vi "CAN Get Error Text.vi"(8 "error in (no error)":errorcluster, 9 "Buffer":string, 10 "Language":u16, 11 "Error":u32) -> (0 "error out":errorcluster, 1 "Buffer out":string, 3 "function return":u32)   [LabVIEW 2025, in "PCAN2023.lvlib"]
doc: "Returns a descriptive text of a given TPCANStatus error code, in any desired language\n\nTPCANStatus __stdcall CAN_GetErrorText(\n TPCANStatus Error, \n WORD Language, \n LPSTR Buffer);"
uses:
  PCAN2023.lvlib
  x64/PCANBasic.dll
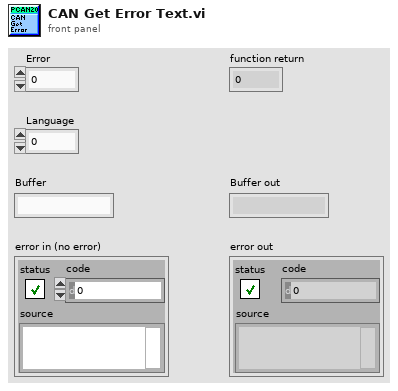
[diagram p1: front panel]
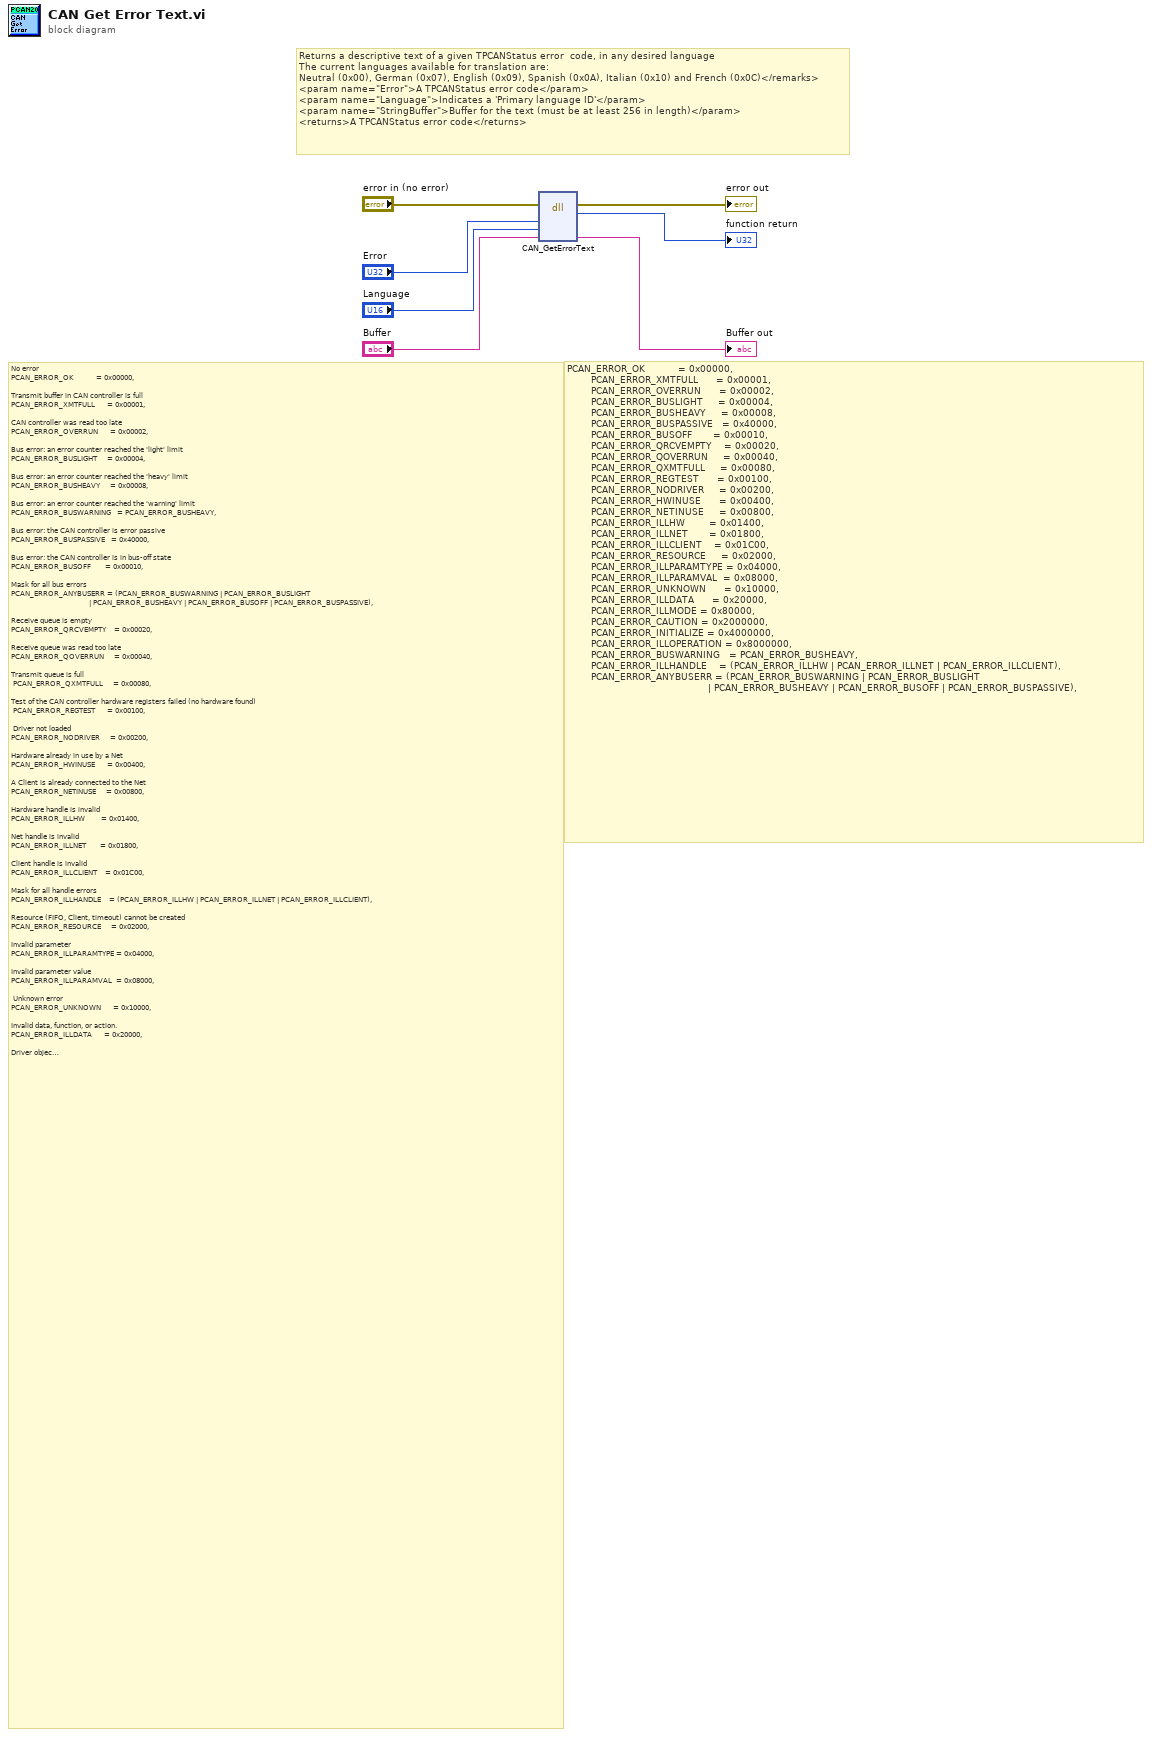
[diagram p0: block diagram]
diagram:
  # "PCAN_ERROR_OK           = 0x00000,\n        PCAN_ERROR_XMTFULL      = 0x00001,\n        PCAN_ERROR_OVERRUN      = 0x00002,  \n        PCAN_ERROR_BUSLIGHT     = 0x00004,  \n        PCAN_ERROR_BUSHEAVY     = 0x00008,  \n        PCAN_ERROR_BUSPASSIVE   = 0x40000,\n        PCAN_ERROR_BUSOFF       = 0x00010,  \n        PCAN_ERROR_QRCVEMPTY    = 0x00020,  \n        PCAN_ERROR_QOVERRUN     = 0x00040,  \n        PCAN_ERROR_QXMTFULL     = 0x00080,  \n        PCAN_ERROR_REGTEST      = 0x00100,\n        PCAN_ERROR_NODRIVER     = 0x00200,\n        PCAN_ERROR_HWINUSE      = 0x00400,\n        PCAN_ERROR_NETINUSE     = 0x00800,\n        PCAN_ERROR_ILLHW        = 0x01400,\n        PCAN_ERROR_ILLNET       = 0x01800,\n        PCAN_ERROR_ILLCLIENT    = 0x01C00,\n        PCAN_ERROR_RESOURCE     = 0x02000,\n        PCAN_ERROR_ILLPARAMTYPE = 0x04000,\n        PCAN_ERROR_ILLPARAMVAL  = 0x08000,\n        PCAN_ERROR_UNKNOWN      = 0x10000,\n        PCAN_ERROR_ILLDATA      = 0x20000,\n        PCAN_ERROR_ILLMODE = 0x80000,\n        PCAN_ERROR_CAUTION = 0x2000000,\n        PCAN_ERROR_INITIALIZE = 0x4000000,\n        PCAN_ERROR_ILLOPERATION = 0x8000000,\n        PCAN_ERROR_BUSWARNING   = PCAN_ERROR_BUSHEAVY,\n        PCAN_ERROR_ILLHANDLE    = (PCAN_ERROR_ILLHW | PCAN_ERROR_ILLNET | PCAN_ERROR_ILLCLIENT),\n        PCAN_ERROR_ANYBUSERR = (PCAN_ERROR_BUSWARNING | PCAN_ERROR_BUSLIGHT \n                                               | PCAN_ERROR_BUSHEAVY | PCAN_ERROR_BUSOFF | PCAN_ERROR_BUSPASSIVE),"
  # "No error\nPCAN_ERROR_OK           = 0x00000,\n\nTransmit buffer in CAN controller is full\nPCAN_ERROR_XMTFULL      = 0x00001,\n\nCAN controller was read too late        \nPCAN_ERROR_OVERRUN      = 0x00002,\n  \nBus error: an error counter reached the 'light' limit\nPCAN_ERROR_BUSLIGHT     = 0x00004,\n  \nBus error: an error counter reached the 'heavy' limit\nPCAN_ERROR_BUSHEAVY     = 0x00008, \n \nBus error: an error counter reached the 'warning' limit\nPCAN_ERROR_BUSWARNING   = PCAN_ERROR_BUSHEAVY,\n\nBus error: the CAN controller is error passive\nPCAN_ERROR_BUSPASSIVE   = 0x40000,\n\nBus error: the CAN controller is in bus-off state\nPCAN_ERROR_BUSOFF       = 0x00010,  \n\nMask for all bus errors\nPCAN_ERROR_ANYBUSERR = (PCAN_ERROR_BUSWARNING | PCAN_ERROR_BUSLIGHT \n                                       | PCAN_ERROR_BUSHEAVY | PCAN_ERROR_BUSOFF | PCAN_ERROR_BUSPASSIVE),\n\nReceive queue is empty\nPCAN_ERROR_QRCVEMPTY    = 0x00020,  \n\nReceive queue was read too late\nPCAN_ERROR_QOVERRUN     = 0x00040,  \n\nTransmit queue is full\n PCAN_ERROR_QXMTFULL     = 0x00080, \n \nTest of the CAN controller hardware registers failed (no hardware found)\n PCAN_ERROR_REGTEST      = 0x00100,\n\n Driver not loaded\nPCAN_ERROR_NODRIVER     = 0x00200,\n\nHardware already in use by a Net\nPCAN_ERROR_HWINUSE      = 0x00400,\n\nA Client is already connected to the Net\nPCAN_ERROR_NETINUSE     = 0x00800,\n\nHardware handle is invalid\nPCAN_ERROR_ILLHW        = 0x01400,\n\nNet handle is invalid\nPCAN_ERROR_ILLNET       = 0x01800,\n\nClient handle is invalid\nPCAN_ERROR_ILLCLIENT    = 0x01C00,\n\nMask for all handle errors\nPCAN_ERROR_ILLHANDLE    = (PCAN_ERROR_ILLHW | PCAN_ERROR_ILLNET | PCAN_ERROR_ILLCLIENT),\n\nResource (FIFO, Client, timeout) cannot be created\nPCAN_ERROR_RESOURCE     = 0x02000,\n\nInvalid parameter\nPCAN_ERROR_ILLPARAMTYPE = 0x04000,\n\nInvalid parameter value\nPCAN_ERROR_ILLPARAMVAL  = 0x08000,\n\n Unknown error\nPCAN_ERROR_UNKNOWN      = 0x10000,\n\nInvalid data, function, or action.\nPCAN_ERROR_ILLDATA      = 0x20000,\n\nDriver object state is wrong for the attempted operation\nPCAN_ERROR_ILLMODE = 0x80000,\n\nAn operation was successfully carried out, however, irregularities were registered\nPCAN_ERROR_CAUTION = 0x2000000,\n\nChannel is not initialized\n        /// <remarks>Value was changed from 0x40000 to 0x4000000</remarks>\nPCAN_ERROR_INITIALIZE = 0x4000000,\n\nInvalid operation\n        /// <remarks>Value was changed from 0x80000 to 0x8000000</remarks>\nPCAN_ERROR_ILLOPERATION = 0x8000000,"
  # "Returns a descriptive text of a given TPCANStatus error  code, in any desired language\nThe current languages available for translation are: \nNeutral (0x00), German (0x07), English (0x09), Spanish (0x0A), Italian (0x10) and French (0x0C)</remarks>\n<param name=\"Error\">A TPCANStatus error code</param>\n<param name=\"Language\">Indicates a 'Primary language ID'</param>\n<param name=\"StringBuffer\">Buffer for the text (must be at least 256 in length)</param>\n<returns>A TPCANStatus error code</returns>"
  n1 = dll-call lib="C:/UTP/LabView/Communication Handle/PCAN2023/x64/PCANBasic.dll" fn="CAN_GetErrorText"(error in="error in (no error)", "Error"="Error", "Language"="Language", "Buffer"="Buffer") -> (error out=→"error out":errorcluster, "return type"=→"function return":u32, "Buffer"=→"Buffer out":string)  [unwired: 4 in, 1 out]
